vi "APN Main.vi"() -> ()   [LabVIEW 2021]
doc: "This template is for the Queued Message Handler design pattern.\n\nThe Event Handling Loop generates messages based on user interface actions.\n\nThe Message Handling Loop processes messages generated by the Event Handling Loop, or by other messages. The messages are string values, so new messages can be added easily to the Message Cases case structure in the Message Handling Loop. Each message cluster can also provide an optional value for Message Data, which is a variant that can be converted to whatever message-specific data is required."
uses:
  8e49a1ec-eeeb-45d9-a73b-170891d0341b.vi
  support/Message Queue/Enqueue Message (Single).vi
  <vilib>/Utility/error.llb/Error Cluster From Error Code.vi
  <vilib>/ErrorRing/Error Ring.xnode
  support/Message Queue/Message Queue.lvlib
  support/User Event - Stop/User Event - Stop.lvlib
panel:
  out "APN REVISION NUMBER":string
  out "GRBL CURRENT CONFIG":string
  out "GRBL VERSION":string
  out "READ BUFFER":string
  in  "Tab Control":T1(tab)
  in  "Apply":bool
  in  "GRBL COM PORT":refnum<visa-resource-name>
  in  "EXTERNAL MICROCONTROLLER":refnum<visa-resource-name>
  in  "Resume":bool
  in  "Start":bool
  in  "Stop":bool
  in  "Pause":bool
  in  "GCode Command":string
  in  "Send GCode Command":bool
  in  "Upload":bool
  in  "GCODE PATH":path caption="Path"
  out "GCODE FILE LOADED":string
  in  "Unlock Alarm":bool
  in  "Go To X Position":bool
  in  "Spindle Speed":i32(slide) min=0 max=100 step=10 scale=0.0..100.0
  in  "Home":bool
  in  "Spindle Off":bool
  in  "Spindle On":bool
  in  "Go To Z Position":bool
  in  "Z Position":dbl
  in  "Go To Y Position":bool
  in  "Y Position":dbl
  in  "X Position":dbl
  in  "Step Amount(mm)":dbl=1.0 caption="Numeric"
  in  "Z-":bool
  in  "Z+":bool
  in  "Y+":bool
  in  "X+":bool
  in  "Y-":bool
  in  "X-":bool
  in  "Apply Config":bool
  in  "Config Cluster":T2={"Step Pulse(uS)"=10, "Step Idel Delay(mS)"=25, "Junction Deviation"=0.01, "Arc Tolerance"=0.002, "Homing Feed"=25.0, "Homing Seek"=1500.0, "Homing Debounce"=250.0, "Homing Pull-Off"=1.0, "Z Steps"=160.0, "X Max Rate"=5000.0, "Y Max Rate"=5000.0, "Max Spindle "=1000.0, "Z Max Rate"=5000.0, "Min Spindle"=0.0, "X Acceleration"=20.0, "Y Acceleration"=20.0, "X Steps"=160.0, "Y Steps"=160.0, "Z Acceleration"=20.0, "X Max Travel"=838.0, "Y Max Travel"=600.0, "Z Max Travel"=300.0, "Step Enable Invert"=enum."Disable", "Limit Pins Invert"=enum."Disable", "Status Report"=enum."Postition Type", "Report Unit"=enum."mm", "Probe Pins Invert"=enum."Disable", "Soft Limits"=enum."Enable", "Hard Limits"=enum."Enable", "Homing Cycle"=enum."Enable", "Homing Invert"=enum."X' Y' Z'", "Laser Mode"=enum."OFF", "Step Port Invert"=enum."X Y Z", "Direction Invert"=enum."X' Y' Z'"}
  in  "STOP":bool
  # "Created By: Brady Barlow, Tyler Tidmore, Lan Duong"
  # "Welcome to the APN application. Use the dropdowns below to setup communication with the APN machine."
  # "Y+"
  # "X-"
  # "X+"
  # "Y-"
  # "Z+"
  # "Z-"
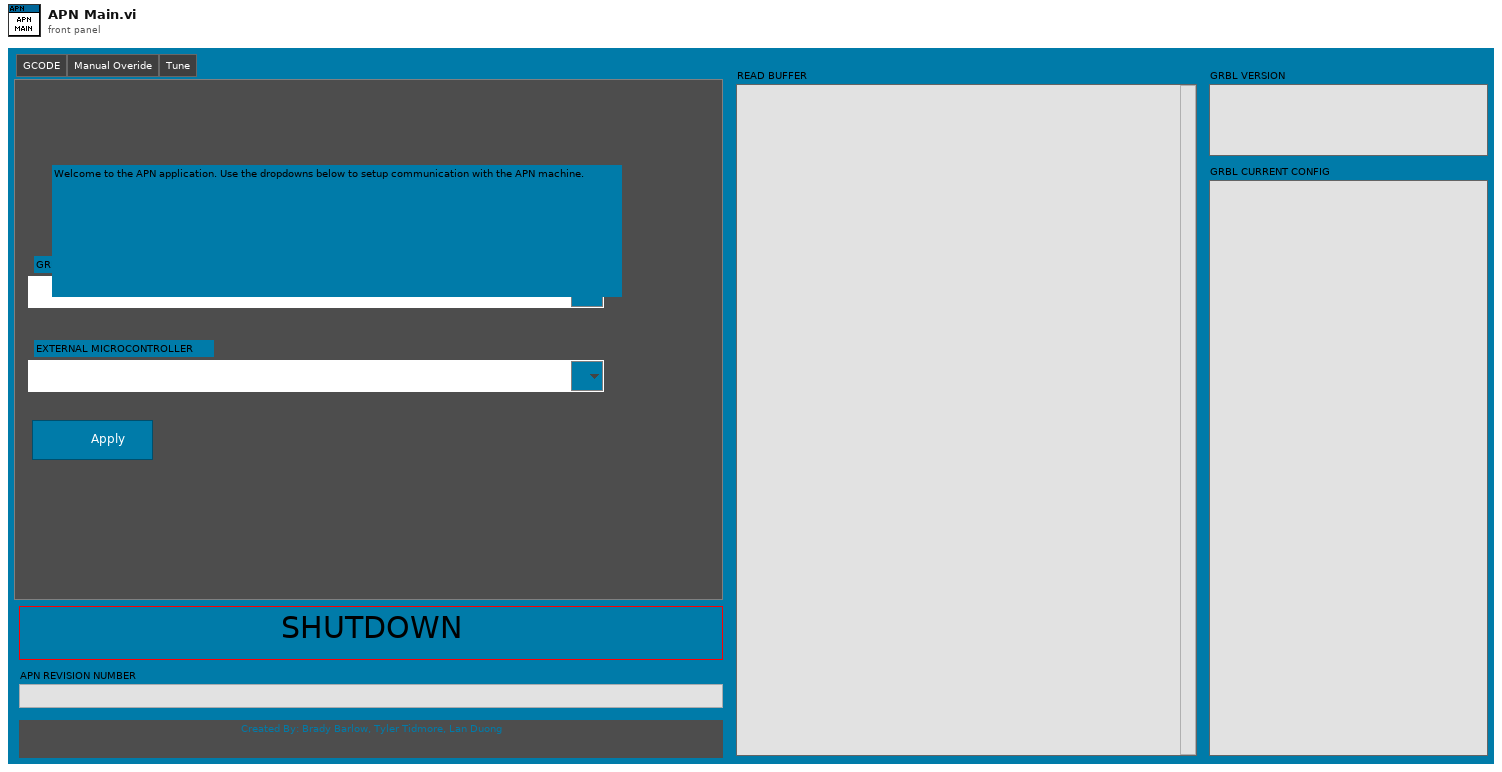
[diagram p1: front panel]
types:
  T1 = enum32{"Serial Configuration", "GCODE", "Manual Overide", "Tune"}
  T2 = cluster{"Step Pulse(uS)":i32, "Step Idel Delay(mS)":i32, "Junction Deviation":dbl, "Arc Tolerance":dbl, "Homing Feed":dbl, "Homing Seek":dbl, "Homing Debounce":dbl, "Homing Pull-Off":dbl, "Z Steps":dbl, "X Max Rate":dbl, "Y Max Rate":dbl, "Max Spindle ":dbl, "Z Max Rate":dbl, "Min Spindle":dbl, "X Acceleration":dbl, "Y Acceleration":dbl, "X Steps":dbl, "Y Steps":dbl, "Z Acceleration":dbl, "X Max Travel":dbl, "Y Max Travel":dbl, "Z Max Travel":dbl, "Step Enable Invert":enum16{"Disable", "Enable"}, "Limit Pins Invert":enum16{"Disable", "Enable"}, "Status Report":enum16{"", "Postition Type", "Buffer Data"}, "Report Unit":enum16{"mm", "Inches"}, "Probe Pins Invert":enum16{"Disable", "Enable"}, "Soft Limits":enum16{"Disable", "Enable"}, "Hard Limits":enum16{"Disable", "Enable"}, "Homing Cycle":enum16{"Disable", "Enable"}, "Homing Invert":enum16{"X Y Z", "X' Y Z", "X Y' Z", "X' Y' Z", "X Y Z'", "X' Y Z'", "X Y' Z'", "X' Y' Z'"}, "Laser Mode":enum16{"OFF", "ON"}, "Step Port Invert":enum16{"X Y Z", "X' Y Z", "X Y' Z", "X' Y' Z", "X Y Z'", "X' Y Z'", "X Y' Z'", "X' Y' Z'"}, "Direction Invert":enum16{"X Y Z", "X' Y Z", "X Y' Z", "X' Y' Z", "X Y Z'", "X' Y Z'", "X Y' Z'", "X' Y' Z'"}}
  T3 = typedef "Message Queue.lvlib/All Message Queues.ctl" = cluster{"UI":refnum<queue>}
  T4 = cluster{"Machine Out":refnum<visa-resource-name>, "EXTERNAL MICROCONTROLLER":refnum<visa-resource-name>}
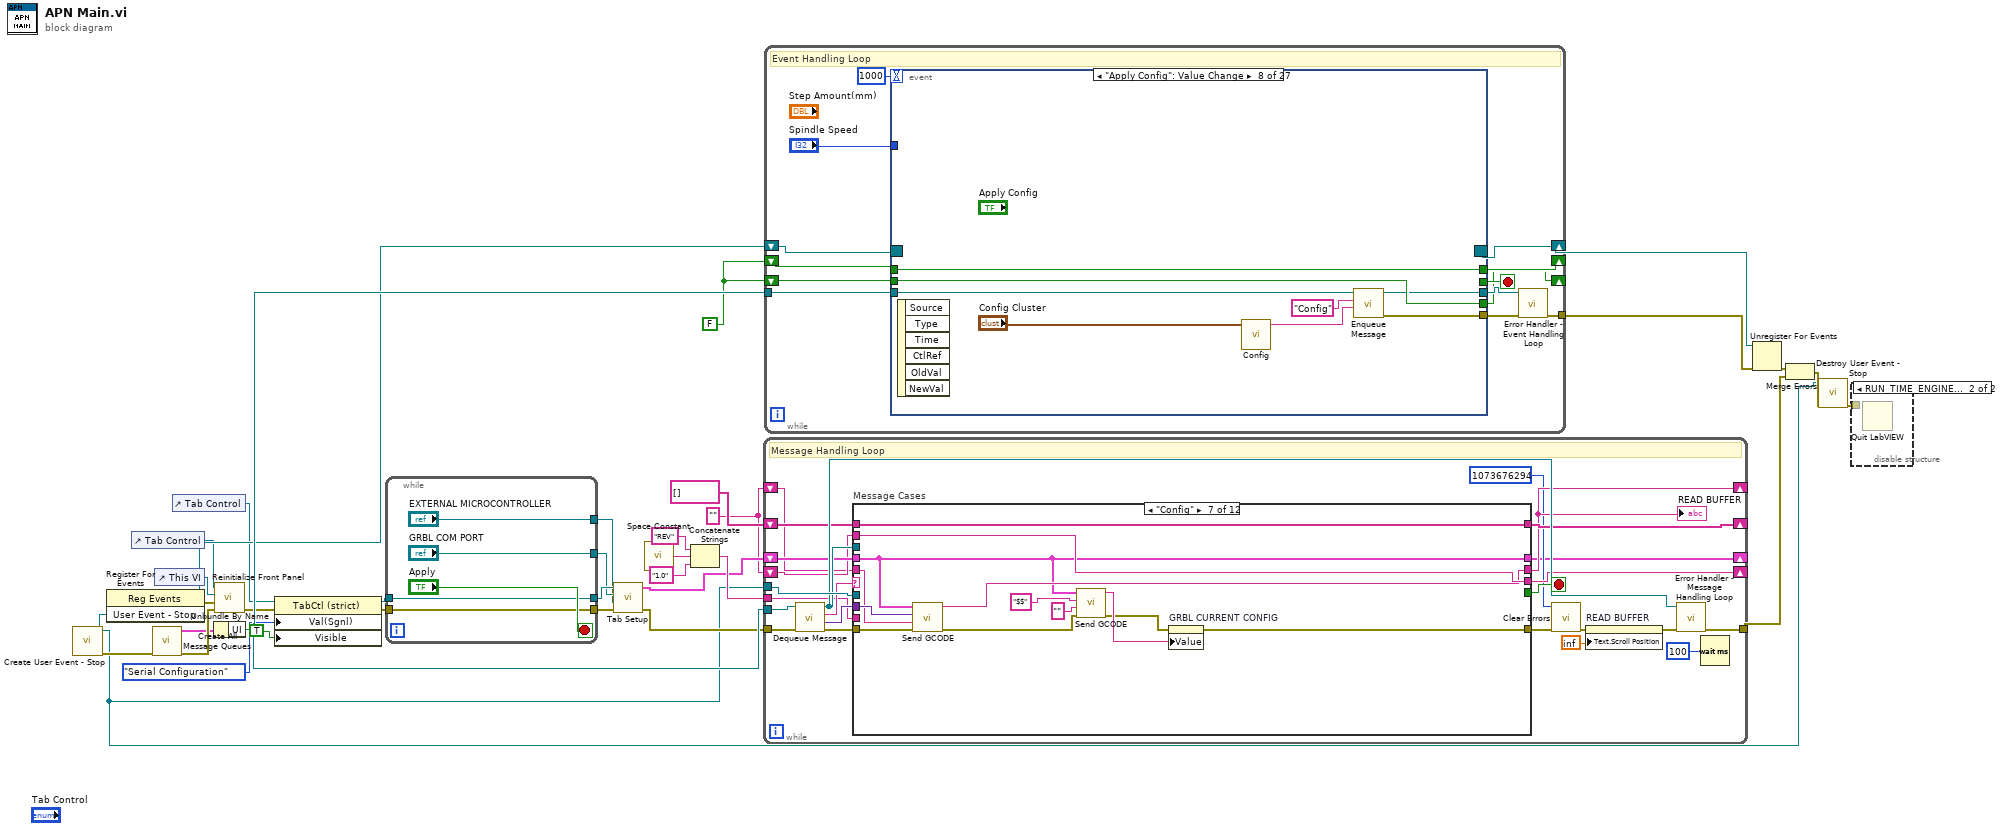
[diagram p0: block diagram]
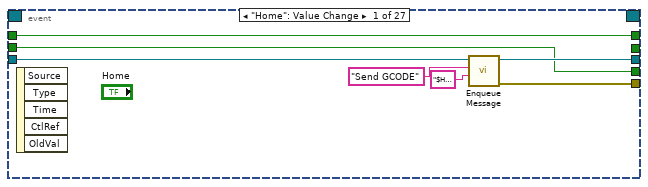
[diagram p3: hidden frame]
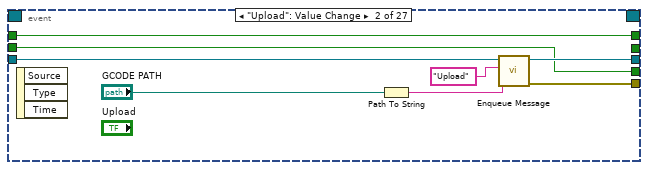
[diagram p4: hidden frame]
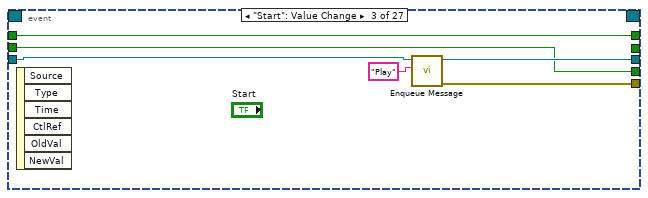
[diagram p5: hidden frame]
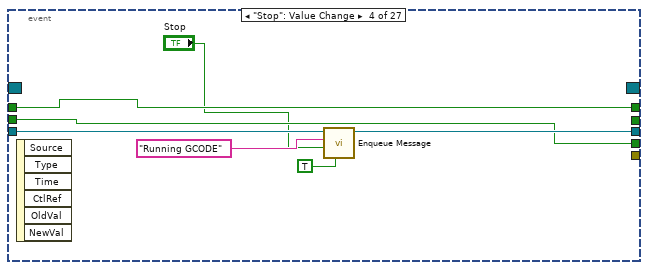
[diagram p6: hidden frame]
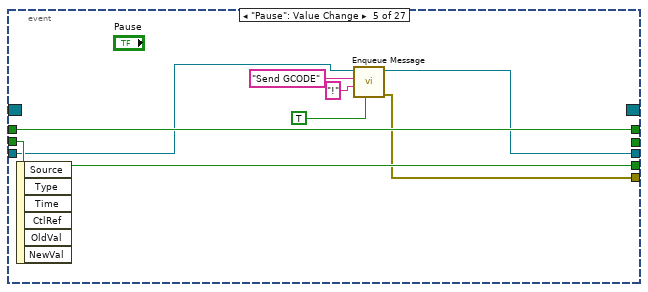
[diagram p7: hidden frame]
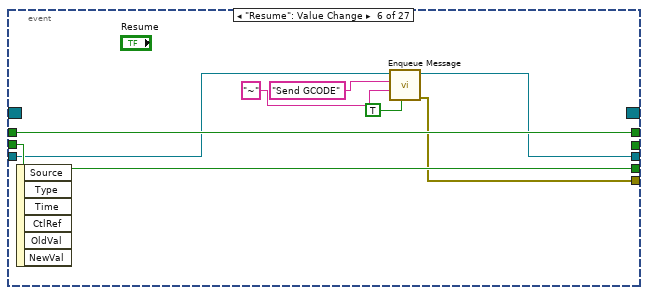
[diagram p8: hidden frame]
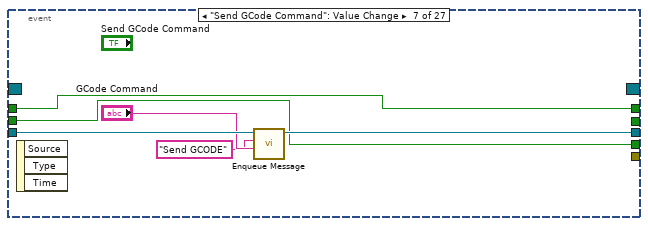
[diagram p9: hidden frame]
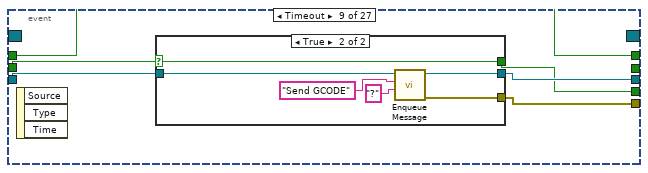
[diagram p10: hidden frame]
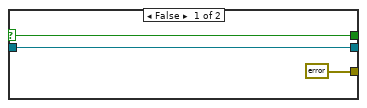
[diagram p11: hidden frame]
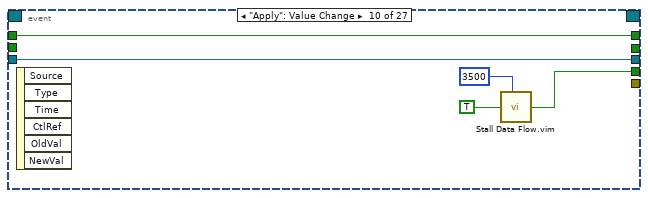
[diagram p12: hidden frame]
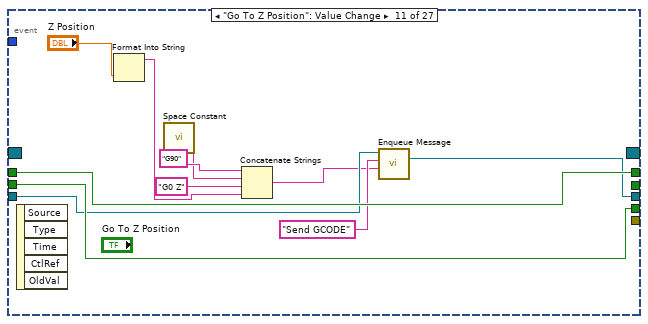
[diagram p13: hidden frame]
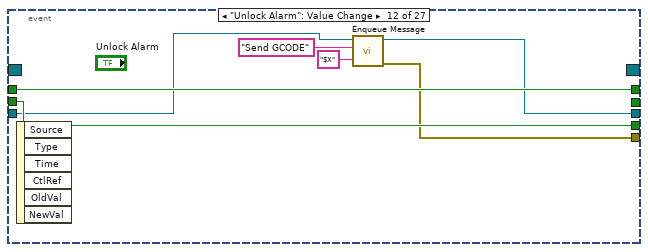
[diagram p14: hidden frame]
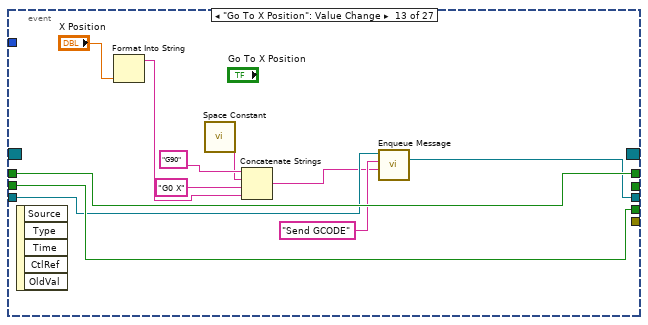
[diagram p15: hidden frame]
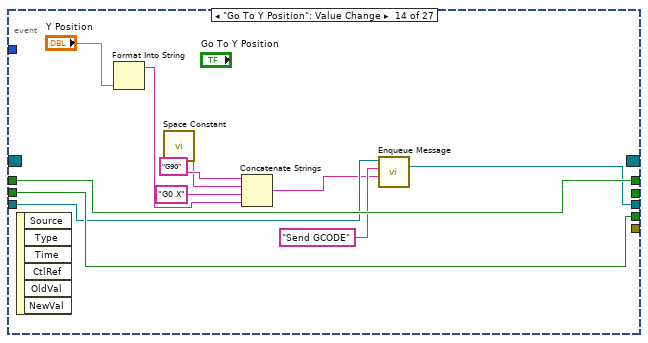
[diagram p16: hidden frame]
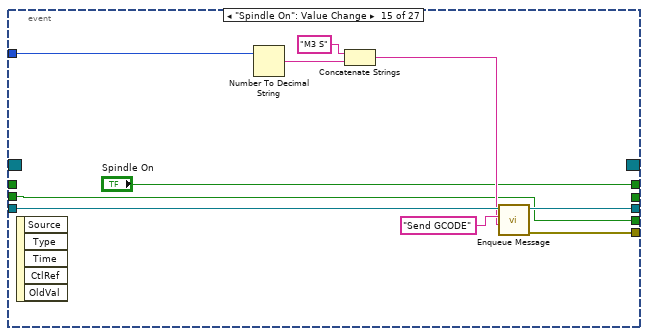
[diagram p17: hidden frame]
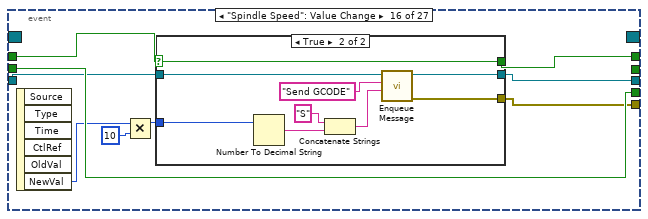
[diagram p18: hidden frame]
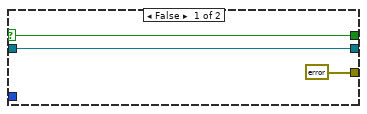
[diagram p19: hidden frame]
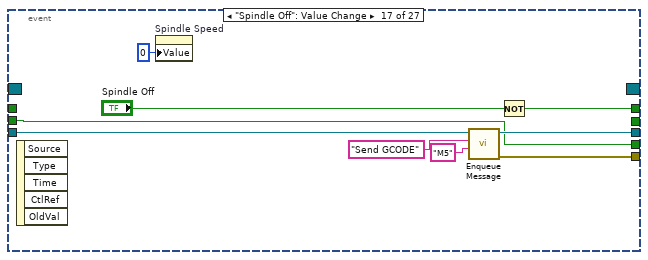
[diagram p20: hidden frame]
diagram:
  w3 = FALSE
  w2 = ""
  n1 = call "Create User Event - Stop.vi"() -> ("error out"=w30:errorcluster, "User Event - Stop"=w1:refnum<user-event>)  [unwired: 10 in]
  n2 = register-events(w1) -> (reference out=w26:refnum<event-registration>, error out=w25:errorcluster)  [unwired: 2 in]
  n3 = control-ref of="Tab Control"() -> (w23:refnum<vi>)
  n4 = call "Create All Message Queues.vi"("error in (no error)"=w30) -> ("error out"=w34:errorcluster, "Message Queues out"=w33:T3)  [unwired: 9 in]
  n5 = control-ref of="This VI"() -> (w24:refnum<vi>)
  n6 = control-ref of="Tab Control"() -> (w15:refnum<vi>)
  n7 = Unbundle By Name(w33) -> ("UI"=w31:refnum<queue>)
  n8 = call "Reinitialize Front Panel.vi"("error in (no error)"=w34, "error in"=w25, "This VI"=w24, "TabControl in"=w23) -> ("error out"=w11:errorcluster)  [unwired: 7 in]
  n9 = property on="Property Node" class="TabCtl (strict)"(reference=w15, error in=w11, "Val(Sgnl)"=T1."Serial Configuration" ("Value (Signaling)"), "Visible"=TRUE) -> (reference out=w12:refnum<vi>, error out=w4:errorcluster)
  n10 = while {
    tunnel: ["GRBL COM PORT"] -> w6
    tunnel: ["EXTERNAL MICROCONTROLLER"] -> w5
    tunnel: w12 -> [w36]
    tunnel: [w36] -> w7
    tunnel: [w35] -> w9
    tunnel: w4 -> [w35]
    stop <- "Apply" stop-if-true
  }
  n11 = call "Tab Setup.vi"("error in (no error)"=w9, "EXTERNAL MICROCONTROLLER"=w5, "GRBL COM PORT"=w6, "TabControl in"=w7) -> ("error out"=w8:errorcluster, "Cluster"=w10:T4)  [unwired: 6 in]
  n12 = call <vilib>:"Space Constant.vi"() -> ("String"=w20:string)
  n13 = Concatenate Strings("REV" ("APN REVISION NUMBER"), w20, "1.0" ("string")) -> (w17:string)
  n14 = while {
    tunnel: w31 -> [w57]
    tunnel: w1 -> [w62]
    tunnel: w8 -> [w61]
    tunnel: [w44] -> w32
    shift-right: [w41] -> _
    shift-left: w10 -> [w55]
    shift-right: [w54] -> _
    shift-left: w2 -> [w53]
    shift-right: [w52] -> _
    shift-left: string[] [] ("G-Code Array out") -> [w51]
    shift-right: [w49] -> _
    shift-left: w2 -> [w48]
    tunnel: w17 -> [w47]
    stop <- w63 stop-if-true
    # "Message Handling Loop"
    n15 = call "Dequeue Message.vi"("error in (no error)"=w61, "Message Queue"=w57) -> ("error out"=w60:errorcluster, "Message Data"=w58:variant, "Message"=w59:string, "dup Message Queue"=w56:refnum<queue>)  [unwired: 6 in]
    n16 = case "Message Cases" shown="\"Config\"" w59 {
      selector: w59 -> [w68 _ _ _ _ _ _ _ _ _ _ _]
      tunnel: w56 -> [_ w80 _ _ w108 _ _ w140 _ _ w171 w190]
      tunnel: w60 -> [_ w77 w91 w98 w109 w117 w130 w137 w149 w164 w174 w178]
      tunnel: [w69 w81 w86 w97 w109 w114 w121 w136 w148 w159 w173 w179] -> w40
      tunnel: [_ _ _ _ _ _ _ _ _ _ _ TRUE] -> w63
      tunnel: w58 -> [_ _ _ w102 _ w118 w131 w143 w150 w163 _ w183]
      tunnel: w62 -> [_ _ _ _ _ _ _ _ _ _ _ w187]
      tunnel: [w67 w78 w87 w99 w110 w115 w126 w138 w152 w158 w168 w176] -> w41
      tunnel: w55 -> [w67 w78 w90 w99 w110 w115 w126 w139 w152 w158 w168 w176]
      tunnel: [w66 w85 w94 w100 w111 w119 w132 w144 w154 w157 w167 w182] -> w54
      tunnel: w53 -> [w66 w85 w94 _ w111 w119 w132 w144 w154 w157 w167 w182]
      tunnel: [w65 w84 w93 w96 w104 w116 w129 w141 w153 w156 w166 w181] -> w52
      tunnel: w51 -> [w65 w84 w93 w96 _ w116 w129 w142 w153 w156 w166 w181]
      tunnel: [w64 w83 w92 w95 w105 w113 w128 w133 w145 w155 w165 w180] -> w49
      tunnel: w48 -> [w64 w83 w92 w95 w105 w112 w127 w135 w146 w155 w165 w180]
      tunnel: w47 -> [_ w79 _ _ _ _ _ _ _ _ _ _]
      frame Default {
        # "'Default' case only runs if there is a message that isn't defined in any of the other cases.  Output a programming error."
        n17 = xnode "Error Ring"("parameter 0"=w68) -> ("error out"=w69:errorcluster)
      }
      frame "Initialize" {
        n18 = call-poly "Enqueue Message.vi"("error in (no error)"=w77, "Message"="GRBL INFO", "Message Queue"=w80) -> ("error out"=w81:errorcluster)  [unwired: 7 in, 1 out]
        "APN REVISION NUMBER" <- w79
      }
      frame "GRBL INFO" {
        n19 = call "GRBL INFO.vi"("error in (no error)"=w91, "Cluster in"=w90) -> ("error out"=w86:errorcluster, "GRBL VERSION"=→"GRBL VERSION":string, "Cluster out"=w87:T4, "GRBL CURRENT CONFIG"=→"GRBL CURRENT CONFIG":string)  [unwired: 6 in]
      }
      frame "Upload" {
        n20 = Variant To Data(error in=w98, type="", Variant=w102) -> (data=w100:string, error out=w97:errorcluster)
        "GCODE FILE LOADED" <- w100
      }
      frame "Play" {
        n21 = String To Path(string=w111) -> (path=w103:path)
        n22 = call-poly "Enqueue Message.vi"("Message Data"=FALSE, "Message"="Running GCODE", "Message Queue"=w108) -> ()  [unwired: 7 in, 2 out]
        n23 = call "File to Gcode.vi"("File Path"=w103) -> ("G-Code Array"=w104:string[])  [unwired: 10 in]
      }
      frame "Send GCODE" {
        n24 = call "Send GCODE.vi"("error in (no error)"=w117, "String in"=w112, "Message Data"=w118, "Cluster"=w115) -> ("error out"=w114:errorcluster, "String out"=w113:string)  [unwired: 6 in]
      }
      frame "Config" {
        n25 = call "Send GCODE.vi"("error in (no error)"=w130, "String in"=w127, "Message Data"=w131, "Cluster"=w126) -> ("error out"=w125:errorcluster, "String out"=w128:string)  [unwired: 6 in]
        n26 = call "Send GCODE.vi"("error in (no error)"=w125, "String in"="", "Message Data"="$$", "Cluster"=w126) -> ("error out"=w122:errorcluster, "String out"=w124:string)  [unwired: 6 in]
        n27 = property on="GRBL CURRENT CONFIG" class="Str"(error in=w122, "Value"=w124) -> (error out=w121:errorcluster)  [unwired: 1 in, 1 out]
      }
      frame "Running GCODE" {
        n28 = call "Running GCODE.vi"("Message Data"=w143, "G-Code Array in"=w142, "error in (no error)"=w137, "Cluster in"=w139, "dup Message Queue"=w140) -> ("error out"=w136:errorcluster, "G-Code Array out"=w141:string[], "String"=w134:string, "Cluster out"=w138:T4)  [unwired: 3 in]
        n29 = Concatenate Strings(w135, w134) -> (w133:string)
      }
      frame "Jog" {
        n30 = Unbundle By Name(w152) -> ("Machine Out"=w151:refnum<visa-resource-name>)
        n31 = call "Jog GCODE.vi"("error in"=w149, "Variant"=w150, "VISA resource name"=w151) -> ("error out"=w148:errorcluster, "String"=w147:string)  [unwired: 7 in]
        n32 = Concatenate Strings(w146, w147) -> (w145:string)
      }
      frame "Error" {
        # "Error - Display an error dialog. This message is sent by the \"Error Handler\" VIs at the end of other loops in this application."
        n33 = Variant To Data(error in=w164, type=errorcluster {"status"=FALSE, "code"=0, "source"=""} ("error constant"), Variant=w163) -> (data=w161:errorcluster, error out=w160:errorcluster)
        n34 = call <vilib>:"Simple Error Handler.vi"("error in (no error)"=w161) -> ()  [unwired: 4 in, 5 out]
        n35 = Merge Errors(w160) -> (w159:errorcluster)
      }
      frame "Confirm Quit" {
        # "Confirm Quit - Message that can confirm whether or not the user wants to exit the application."
        n36 = call-poly "Enqueue Message.vi"("Priority Message? (F)"=TRUE, "error in (no error)"=w174, "Message"="Exit", "Message Queue"=w171) -> ("error out"=w172:errorcluster)  [unwired: 6 in, 1 out]
        n37 = Merge Errors(w172) -> (w173:errorcluster)
      }
      frame "Exit" {
        # "Exit - Exit the application."
        n38 = Unbundle By Name(w176) -> ("Machine Out"=w175:refnum<visa-resource-name>)
        n39 = Variant To Data(type=errorcluster {"status"=FALSE, "code"=0, "source"=""} ("error constant"), Variant=w183) -> (data=w184:errorcluster)  [unwired: 1 in, 1 out]
        n40 = call <vilib>:"Simple Error Handler.vi"("error in (no error)"=w184) -> ()  [unwired: 4 in, 5 out]
        n41 = VISA Close(VISA resource name=w175, error in (no error)=w178) -> (error out=w177:errorcluster)
        n42 = call "Fire User Event - Stop.vi"("User Event - Stop"=w187) -> ("error out"=w186:errorcluster)  [unwired: 10 in]
        n43 = Release Queue(queue=w190, error in (no error)=w177) -> (error out=w188:errorcluster)  [unwired: 1 in, 2 out]
        n44 = Merge Errors(w186, w188) -> (w179:errorcluster)
      }
    }
    "READ BUFFER" <- w49
    n45 = call <vilib>:"Clear Errors.vi"("error in (no error)"=w40, "specific error code to clear (0: all)"=1073676294) -> ("error out"=w43:errorcluster)  [unwired: 4 in, 1 out]
    n46 = property on="READ BUFFER" class="Str"(error in=w43, "Text.Scroll Position"=inf) -> (error out=w42:errorcluster)  [unwired: 1 in, 1 out]
    n47 = call "Error Handler - Message Handling Loop.vi"("error in (no error)"=w42, "Message Queue"=w56) -> ("dup error in"=w44:errorcluster)  [unwired: 8 in, 1 out]
    n48 = Wait (ms)(milliseconds to wait=u32 100) -> ()  [unwired: 1 out]
  }
  n49 = while {
    tunnel: w31 -> [w203]
    shift-right: [w201] -> w28
    shift-left: w26 -> [w202]
    tunnel: [w197] -> w27
    shift-right: [w196] -> _
    shift-left: w3 -> [w195]
    shift-right: [w193] -> _
    shift-left: w3 -> [w192]
    stop <- w199 stop-if-true
    # "Event Handling Loop"
    n50 = event shown="[7] \"Apply Config\": Value Change" {
      selector: w202 -> [_ _ _ _ _ _ _ _ _ _ _ _ _ _ _ _ _ _ _ _ _ _ _ _ _ _ _]
      dyn-events: [_ _ _ _ _ _ _ _ _ _ _ _ _ _ _ _ _ _ _ _ _ _ _ _ _ _ _] -> w201
      timeout: 1000 -> [_ _ _ _ _ _ _ _ _ _ _ _ _ _ _ _ _ _ _ _ _ _ _ _ _ _ _]
      tunnel: [_ _ _ _ _ _ _ _ _ _ _ _ _ _ _ _ _ _ _ _ _ _ _ _ TRUE ("Discard?") _ _] -> w199
      tunnel: w203 -> [w210 w218 w223 w230 w234 w242 w253 w258 w266 w281 w285 w295 w304 w314 w329 w337 w359 w369 w377 w385 w393 w401 w409 w416 w420 w423 w430]
      tunnel: [w206 w216 w222 _ w235 w243 _ w255 w264 _ _ w294 _ _ w326 w336 w357 _ _ _ _ _ _ w415 _ _ w429] -> w200
      tunnel: [w207 w217 w221 w229 w233 w241 w249 w257 w265 w281 w284 w293 w303 w313 w328 w338 w360 w368 w376 w384 w392 w400 w408 w414 w420 w423 w428] -> w198
      tunnel: [w205 w212 w220 w227 w239 w247 w250 w261 w267 w280 w292 w299 w310 w321 "Spindle On" w335 w355 w364 w372 w380 w388 w396 w404 w411 w418 w422 w425] -> w196
      tunnel: w195 -> [w205 w212 w220 w227 w239 w247 w250 w261 w267 w280 w292 w299 w310 w321 _ w339 _ w364 w372 w380 w388 w396 w404 w411 w418 w422 w425]
      tunnel: [w204 w211 w219 w226 w238 w246 w248 w260 w262 w278 w291 w298 w309 w320 w324 w340 w354 w363 w371 w379 w387 w395 w403 w410 w417 w421 w424] -> w193
      tunnel: w192 -> [w204 w211 w219 w226 w238 w246 w248 w260 w263 _ w291 w298 w309 w320 w324 w340 w354 w363 w371 w379 w387 w395 w403 w410 w417 w421 w424]
      tunnel: "Spindle Speed" -> [_ _ _ _ _ _ _ _ _ _ _ _ _ _ w322 _ _ _ _ _ _ _ _ _ _ _ _]
      event "Home": Value Change {
        n51 = event-data() -> ()  [unwired: 1 in, 5 out]
        n52 = call-poly "Enqueue Message.vi"("Message Data"="$H\nG10 P0 L20 X0 Y0 Z0\n", "Message"="Send GCODE", "Message Queue"=w210) -> ("error out"=w206:errorcluster, "dup Message Queue"=w207:refnum<queue>)  [unwired: 7 in]
      }
      event "Upload": Value Change {
        n53 = event-data() -> ()  [unwired: 1 in, 3 out]
        n54 = Path To String(path="GCODE PATH") -> (string=w215:string)
        n55 = call-poly "Enqueue Message.vi"("Message Data"=w215, "Message"="Upload", "Message Queue"=w218) -> ("error out"=w216:errorcluster, "dup Message Queue"=w217:refnum<queue>)  [unwired: 7 in]
      }
      event "Start": Value Change {
        n56 = event-data() -> ()  [unwired: 1 in, 6 out]
        n57 = call-poly "Enqueue Message.vi"("Message"="Play", "Message Queue"=w223) -> ("error out"=w222:errorcluster, "dup Message Queue"=w221:refnum<queue>)  [unwired: 8 in]
      }
      event "Stop": Value Change {
        n58 = event-data() -> ()  [unwired: 1 in, 6 out]
        n59 = call-poly "Enqueue Message.vi"("Priority Message? (F)"=TRUE, "Message Data"="Stop", "Message"="Running GCODE", "Message Queue"=w230) -> ("dup Message Queue"=w229:refnum<queue>)  [unwired: 6 in, 1 out]
      }
      event "Pause": Value Change {
        n60 = event-data() -> ()  [unwired: 1 in, 6 out]
        n61 = call-poly "Enqueue Message.vi"("Priority Message? (F)"=TRUE, "Message Data"="!" ("Message"), "Message"="Send GCODE", "Message Queue"=w234) -> ("error out"=w235:errorcluster, "dup Message Queue"=w233:refnum<queue>)  [unwired: 6 in]
      }
      event "Resume": Value Change {
        n62 = event-data() -> ()  [unwired: 1 in, 6 out]
        n63 = call-poly "Enqueue Message.vi"("Priority Message? (F)"=TRUE, "Message Data"="~" ("Message"), "Message"="Send GCODE", "Message Queue"=w242) -> ("error out"=w243:errorcluster, "dup Message Queue"=w241:refnum<queue>)  [unwired: 6 in]
      }
      event "Send GCode Command": Value Change {
        n64 = event-data() -> ()  [unwired: 1 in, 3 out]
        n65 = call-poly "Enqueue Message.vi"("Message Data"="GCode Command", "Message"="Send GCODE", "Message Queue"=w253) -> ("dup Message Queue"=w249:refnum<queue>)  [unwired: 7 in, 1 out]
      }
      event "Apply Config": Value Change {
        n66 = event-data() -> ()  [unwired: 1 in, 6 out]
        n67 = call "Config.vi"("Config Cluster"="Config Cluster") -> ("concatenated string"=w256:string)  [unwired: 10 in]
        n68 = call-poly "Enqueue Message.vi"("Message Data"=w256, "Message"="Config", "Message Queue"=w258) -> ("error out"=w255:errorcluster, "dup Message Queue"=w257:refnum<queue>)  [unwired: 7 in]
      }
      event Timeout {
        n69 = event-data() -> ()  [unwired: 1 in, 3 out]
        n70 = case shown="True" w263 {
          selector: w263 -> [w268 w271]
          tunnel: w266 -> [w270 w274]
          tunnel: [w270 w273] -> w265
          tunnel: [errorcluster {"status"=FALSE, "code"=0, "source"=""} ("error out") w272] -> w264
          tunnel: [w268 w271] -> w262
          frame False {
          }
          frame True {
            n71 = call-poly "Enqueue Message.vi"("Message Data"="?", "Message"="Send GCODE", "Message Queue"=w274) -> ("error out"=w272:errorcluster, "dup Message Queue"=w273:refnum<queue>)  [unwired: 7 in]
          }
        }
      }
      event "Apply": Value Change {
        n72 = event-data() -> ()  [unwired: 1 in, 6 out]
        n73 = call "Stall Data Flow.vim"("value in"=TRUE, "milliseconds to wait"=u32 3500) -> ("value out"=w278:bool)  [unwired: 1 out]
      }
      event "Go To Z Position": Value Change {
        n74 = event-data() -> ()  [unwired: 1 in, 5 out]
        n75 = Format Into String("Z Position") -> (resulting string=w287:string)  [unwired: 3 in, 1 out]
        n76 = call <vilib>:"Space Constant.vi"() -> ("String"=w289:string)
        n77 = Concatenate Strings("G90" ("string"), w289, "G0 Z" ("string"), w287) -> (w283:string)
        n78 = call-poly "Enqueue Message.vi"("Message Data"=w283, "Message"="Send GCODE", "Message Queue"=w285) -> ("dup Message Queue"=w284:refnum<queue>)  [unwired: 7 in, 1 out]
      }
      event "Unlock Alarm": Value Change {
        n79 = event-data() -> ()  [unwired: 1 in, 6 out]
        n80 = call-poly "Enqueue Message.vi"("Message Data"="$X", "Message"="Send GCODE", "Message Queue"=w295) -> ("error out"=w294:errorcluster, "dup Message Queue"=w293:refnum<queue>)  [unwired: 7 in]
      }
      event "Go To X Position": Value Change {
        n81 = event-data() -> ()  [unwired: 1 in, 5 out]
        n82 = Format Into String("X Position") -> (resulting string=w306:string)  [unwired: 3 in, 1 out]
        n83 = call <vilib>:"Space Constant.vi"() -> ("String"=w301:string)
        n84 = Concatenate Strings("G90" ("string"), w301, "G0 X" ("string"), w306) -> (w302:string)
        n85 = call-poly "Enqueue Message.vi"("Message Data"=w302, "Message"="Send GCODE", "Message Queue"=w304) -> ("dup Message Queue"=w303:refnum<queue>)  [unwired: 7 in, 1 out]
      }
      event "Go To Y Position": Value Change {
        n86 = event-data() -> ()  [unwired: 1 in, 6 out]
        n87 = Format Into String("Y Position") -> (resulting string=w316:string)  [unwired: 3 in, 1 out]
        n88 = call <vilib>:"Space Constant.vi"() -> ("String"=w318:string)
        n89 = Concatenate Strings("G90" ("string"), w318, "G0 X" ("string"), w316) -> (w312:string)
        n90 = call-poly "Enqueue Message.vi"("Message Data"=w312, "Message"="Send GCODE", "Message Queue"=w314) -> ("dup Message Queue"=w313:refnum<queue>)  [unwired: 7 in, 1 out]
      }
      event "Spindle On": Value Change {
        n91 = event-data() -> ()  [unwired: 1 in, 5 out]
        n92 = Number To Decimal String(number=w322) -> (decimal integer string=w323:string)  [unwired: 1 in]
        n93 = Concatenate Strings("M3 S", w323) -> (w327:string)
        n94 = call-poly "Enqueue Message.vi"("Message Data"=w327, "Message"="Send GCODE", "Message Queue"=w329) -> ("error out"=w326:errorcluster, "dup Message Queue"=w328:refnum<queue>)  [unwired: 7 in]
      }
      event "Spindle Speed": Value Change {
        n95 = event-data() -> ("NewVal"=w332:i32)  [unwired: 1 in, 5 out]
        n96 = Multiply(x=w332, y=10) -> (x*y=w333:i32)
        n97 = case shown="True" w339 {
          selector: w339 -> [w341 w345]
          tunnel: w333 -> [_ w344]
          tunnel: w337 -> [w343 w348]
          tunnel: [w343 w347] -> w338
          tunnel: [errorcluster {"status"=FALSE, "code"=0, "source"=""} ("error out") w346] -> w336
          tunnel: [w341 w345] -> w335
          frame False {
          }
          frame True {
            n98 = Number To Decimal String(number=w344) -> (decimal integer string=w349:string)  [unwired: 1 in]
            n99 = Concatenate Strings("S", w349) -> (w350:string)
            n100 = call-poly "Enqueue Message.vi"("Message Data"=w350, "Message"="Send GCODE", "Message Queue"=w348) -> ("error out"=w346:errorcluster, "dup Message Queue"=w347:refnum<queue>)  [unwired: 7 in]
          }
        }
      }
      event "Spindle Off": Value Change {
        n101 = event-data() -> ()  [unwired: 1 in, 5 out]
        n102 = property on="Spindle Speed" class="Slide (strict)"("Value"=0 ("Spindle Speed")) -> ()  [unwired: 2 in, 2 out]
        n103 = call-poly "Enqueue Message.vi"("Message Data"="M5" ("Write Buffer"), "Message"="Send GCODE", "Message Queue"=w359) -> ("error out"=w357:errorcluster, "dup Message Queue"=w360:refnum<queue>)  [unwired: 7 in]
        n104 = Not(x="Spindle Off") -> (.not. x?=w355:bool)
      }
      event "X+": Value Change {
        n105 = event-data() -> ()  [unwired: 1 in, 5 out]
        n106 = property on="Step Amount(mm)" class="DigNum (strict)"() -> ("Value"=w362:dbl)  [unwired: 2 in, 2 out]
        n107 = call "Jog.vi"("Direction"="X+", "Step Amount"=w362) -> ("Array"=w366:string[])  [unwired: 8 in]
        n108 = call-poly "Enqueue Message.vi"("Message Data"=w366, "Message"="Jog", "Message Queue"=w369) -> ("dup Message Queue"=w368:refnum<queue>)  [unwired: 7 in, 1 out]
      }
      event "X-": Value Change {
        n109 = event-data() -> ()  [unwired: 1 in, 5 out]
        n110 = property on="Step Amount(mm)" class="DigNum (strict)"() -> ("Value"=w370:dbl)  [unwired: 2 in, 2 out]
        n111 = call "Jog.vi"("Direction"="X-", "Step Amount"=w370) -> ("Array"=w374:string[])  [unwired: 8 in]
        n112 = call-poly "Enqueue Message.vi"("Message Data"=w374, "Message"="Jog", "Message Queue"=w377) -> ("dup Message Queue"=w376:refnum<queue>)  [unwired: 7 in, 1 out]
      }
      event "Y+": Value Change {
        n113 = event-data() -> ()  [unwired: 1 in, 5 out]
        n114 = property on="Step Amount(mm)" class="DigNum (strict)"() -> ("Value"=w378:dbl)  [unwired: 2 in, 2 out]
        n115 = call "Jog.vi"("Direction"="Y+", "Step Amount"=w378) -> ("Array"=w381:string[])  [unwired: 8 in]
        n116 = call-poly "Enqueue Message.vi"("Message Data"=w381, "Message"="Jog", "Message Queue"=w385) -> ("dup Message Queue"=w384:refnum<queue>)  [unwired: 7 in, 1 out]
      }
      event "Y-": Value Change {
        n117 = event-data() -> ()  [unwired: 1 in, 5 out]
        n118 = property on="Step Amount(mm)" class="DigNum (strict)"() -> ("Value"=w386:dbl)  [unwired: 2 in, 2 out]
        n119 = call "Jog.vi"("Direction"="Y-", "Step Amount"=w386) -> ("Array"=w389:string[])  [unwired: 8 in]
        n120 = call-poly "Enqueue Message.vi"("Message Data"=w389, "Message"="Jog", "Message Queue"=w393) -> ("dup Message Queue"=w392:refnum<queue>)  [unwired: 7 in, 1 out]
      }
      event "Z+": Value Change {
        n121 = event-data() -> ()  [unwired: 1 in, 5 out]
        n122 = property on="Step Amount(mm)" class="DigNum (strict)"() -> ("Value"=w394:dbl)  [unwired: 2 in, 2 out]
        n123 = call "Jog.vi"("Direction"="Z+", "Step Amount"=w394) -> ("Array"=w398:string[])  [unwired: 8 in]
        n124 = call-poly "Enqueue Message.vi"("Message Data"=w398, "Message"="Jog", "Message Queue"=w401) -> ("dup Message Queue"=w400:refnum<queue>)  [unwired: 7 in, 1 out]
      }
      event "Z-": Value Change {
        n125 = event-data() -> ()  [unwired: 1 in, 5 out]
        n126 = property on="Step Amount(mm)" class="DigNum (strict)"() -> ("Value"=w402:dbl)  [unwired: 2 in, 2 out]
        n127 = call "Jog.vi"("Direction"="Z-", "Step Amount"=w402) -> ("Array"=w406:string[])  [unwired: 8 in]
        n128 = call-poly "Enqueue Message.vi"("Message Data"=w406, "Message"="Jog", "Message Queue"=w409) -> ("dup Message Queue"=w408:refnum<queue>)  [unwired: 7 in, 1 out]
      }
      event "STOP": Value Change {
        n129 = event-data() -> ()  [unwired: 1 in, 1 out]
        n130 = call-poly "Enqueue Message.vi"("Priority Message? (F)"=TRUE, "Message"="Exit", "Message Queue"=w416) -> ("error out"=w415:errorcluster, "dup Message Queue"=w414:refnum<queue>)  [unwired: 7 in]
      }
      event User Event {
        n131 = event-data() -> ()  [unwired: 1 in, 1 out]
      }
      event Application Instance Close {
        n132 = event-data() -> ()  [unwired: 1 in, 1 out]
      }
      event Panel Close? {
        w426 = TRUE ("Priority Message? (F)")
        n133 = event-data() -> ()  [unwired: 1 in, 1 out]
        n134 = call-poly "Enqueue Message.vi"("Priority Message? (F)"=w426, "Message"="Confirm Quit", "Message Queue"=w430) -> ("error out"=w429:errorcluster, "dup Message Queue"=w428:refnum<queue>)  [unwired: 7 in]
        n135 = event-data("Discard?"=w426) -> ()  [unwired: 1 in, 1 out]
      }
    }
    n136 = call "Error Handler - Event Handling Loop.vi"("error in (no error)"=w200, "Message Queue"=w198) -> ("dup error in"=w197:errorcluster)  [unwired: 8 in, 1 out]
  }
  n137 = Unregister For Events(event registration refnum=w28, error in=w27) -> (error out=w29:errorcluster)
  n138 = Merge Errors(w29, w32) -> (w16:errorcluster)
  n139 = call "Destroy User Event - Stop.vi"("error in (no error)"=w16, "User Event - Stop"=w1) -> ("error out"=w22:errorcluster)  [unwired: 9 in]
  n140 = disable-structure shown="RUN_TIME_ENGINE==True" {
    disable-tunnel: w22 -> [_ _]
    frame condition #0 (active) {
    }
    frame condition #1 {
      n141 = Quit LabVIEW() -> ()  [unwired: 1 in]
    }
  }
